vi "Set IP Subnet Gateway.vi"(8 "Error In":errorcluster, 11 "NIC Info":T1) -> (0 "Error Out":errorcluster, 3 "NIC Info":T1)   [LabVIEW 2014, in "LMH-LINX.lvlib"]
uses:
  <vilib>/MakerHub/LINX/LMH-LINX.lvlib
  <vilib>/MakerHub/LINX/Private/Utilties/Target Management/NIC Info.ctl
  <vilib>/MakerHub/LINX/Private/Utilties/Target Management/NIC Mode.ctl
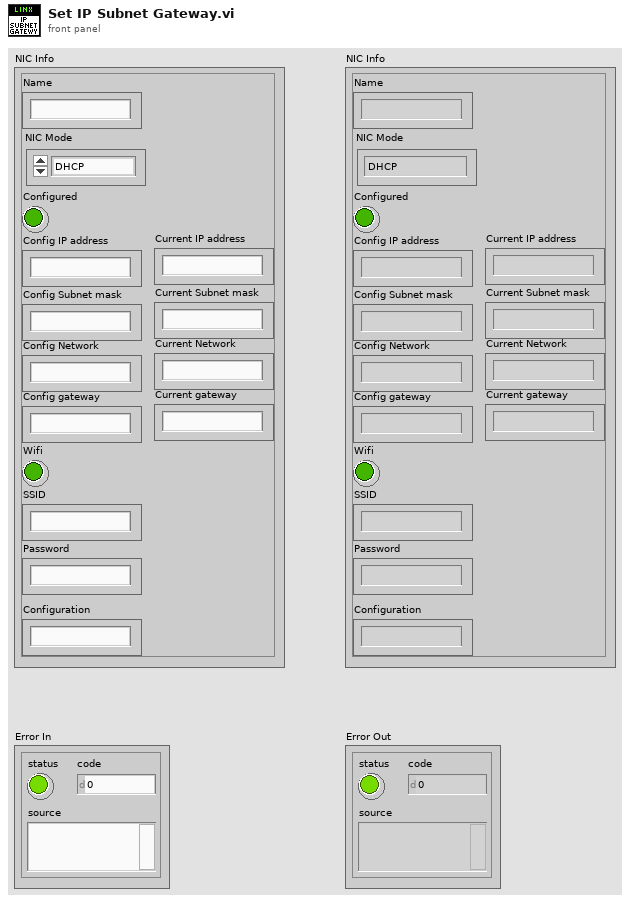
[diagram p1: front panel]
types:
  T1 = typedef "LMH-LINX.lvlib/NIC Info.ctl" = cluster{"Name":string, "NIC Mode":T2, "Configured":bool, "Config IP address":string, "Config Subnet mask":string, "Config Network":string, "Config gateway":string, "Wifi":bool, "SSID":string, "Password":string, "Configuration":string, "Current IP address":string, "Current Subnet mask":string, "Current gateway":string, "Current Network":string}
  T2 = typedef "LMH-LINX.lvlib/NIC Mode.ctl" = enum16{"DHCP", "Static", "Loopback"}
  T3 = typedef "LMH-LINX.lvlib/Network Settings Ctrl Refs.ctl" = cluster{"Hostname":refnum<vi>, "IP address":refnum<vi>, "Subnet mask":refnum<vi>, "Default Gateway":refnum<vi>, "SSID":refnum<vi>, "Password":refnum<vi>, "NIC Status":refnum<vi>, "Network Interface":refnum<vi>, "DCHP":refnum<vi>}
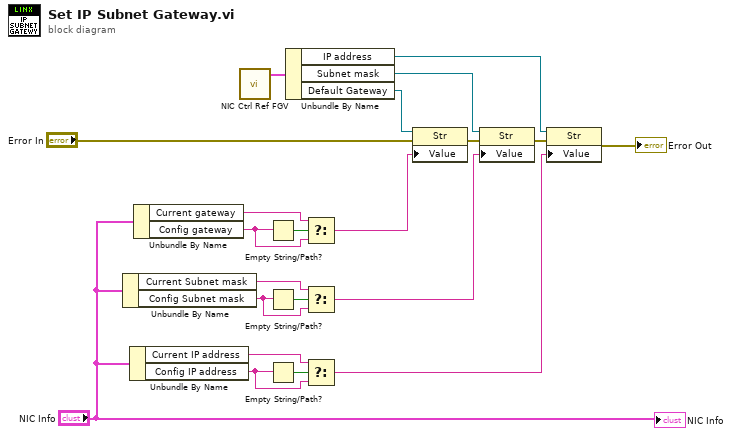
[diagram p0: block diagram]
diagram:
  n1 = Unbundle By Name("NIC Info") -> ("Current Subnet mask"=w8:string, "Config Subnet mask"=w9:string)
  n2 = Unbundle By Name("NIC Info") -> ("Current IP address"=w15:string, "Config IP address"=w14:string)
  n3 = Unbundle By Name("NIC Info") -> ("Current gateway"=w5:string, "Config gateway"=w4:string)
  n4 = call <vilib>:"NIC Ctrl Ref FGV.vi"() -> ("Network Settings Ctrl Refs"=w17:T3)  [unwired: 4 in]
  n5 = Empty String/Path?(string/path=w4) -> (empty?=w6:bool)
  n6 = Empty String/Path?(string/path=w9) -> (empty?=w7:bool)
  n7 = Empty String/Path?(string/path=w14) -> (empty?=w16:bool)
  n8 = Unbundle By Name(w17) -> ("IP address"=w11:refnum<vi>, "Subnet mask"=w12:refnum<vi>, "Default Gateway"=w13:refnum<vi>)
  n9 = Select(t=w5, s=w6, f=w4) -> (s? t:f=w2:string)
  n10 = Select(t=w8, s=w7, f=w9) -> (s? t:f=w3:string)
  n11 = Select(t=w15, s=w16, f=w14) -> (s? t:f=w10:string)
  n12 = property class="Str"(reference=w13, error in="Error In", "Value"=w2) -> (error out=w18:errorcluster)  [unwired: 1 out]
  n13 = property class="Str"(reference=w12, error in=w18, "Value"=w3) -> (error out=w19:errorcluster)  [unwired: 1 out]
  n14 = property class="Str"(reference=w11, error in=w19, "Value"=w10) -> (error out=→"Error Out":errorcluster)  [unwired: 1 out]
  "NIC Info" <- "NIC Info"
